vi "Tusk.GetName (Global).vi"(8 "error in (no error)":errorcluster, 11 "Tusk in":refnum<class "Tusk.lvclass">) -> (0 "error out":errorcluster, 2 "Name(Global)":string, 3 "Tusk out":refnum<class "Tusk.lvclass">)   [LabVIEW 2018, in "Application.lvlib" / "Tusk.lvclass"]
uses:
  Tusk.lvclass
  Tusk.lvclass/Tusk.ctl
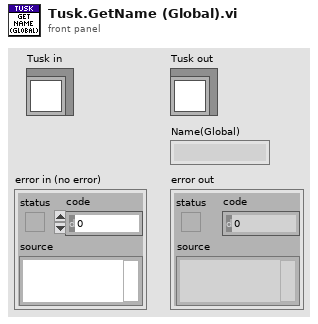
[diagram p1: front panel]
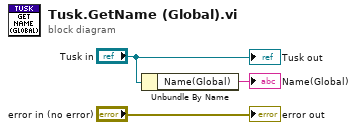
[diagram p0: block diagram]
diagram:
  n1 = Unbundle By Name("Tusk in") -> ("Name(Global)"=→"Name(Global)":string)
  "error out" <- "error in (no error)"
  "Tusk out" <- "Tusk in"
